vi "Check Variant Type.vi"(8 "error in (no error)":errorcluster, 10 "Variant":variant, 11 "Numeric Value in":refnum<class "Numeric Value.lvclass">) -> (0 "error out":errorcluster, 3 "Numeric Value out":refnum<class "Numeric Value.lvclass">)   [LabVIEW 2020, in "Composed Columns.lvlib" / "Numeric Value.lvclass"]
uses:
  Numeric Value.lvclass
  <vilib>/Utility/Data Type/NI_Data Type.lvlib
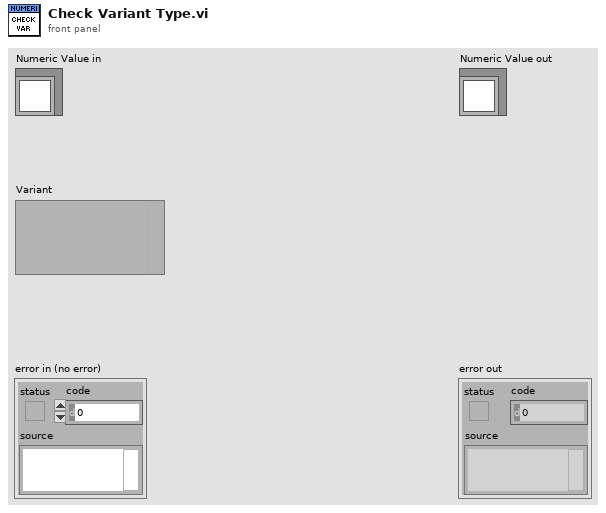
[diagram p1: front panel]
types:
  T1 = typedef "NI_Data Type.lvlib/Data Type.ctl" = enum8{"Invalid Type", "Void", "I8", "I16", "I32", "I64", "U8", "U16", "U32", "U64", "Single Float", "Double Float", "Extended Float", "Single Complex", "Double Complex", "Extended Complex", "Enum U8", "Enum U16", "Enum U32", "Enum U64", "Single Float With Unit", "Double Float With Unit", "Extended Float With Unit", "Single Complex with Unit", "Double Complex with Unit", "Extended Complex with Unit", "Boolean", "String", "Path", "Picture", "Tag", "Array", "Cluster", "Variant", "LV Variant", "Waveform", "Timestamp", "Digital Waveform", "Digital Data", "ExpressData", "Refnum", "External Data", "VI", "Poly VI", "LabVIEW Class Instance", "Fixed Point", "Set Collection", "Map Collection"}
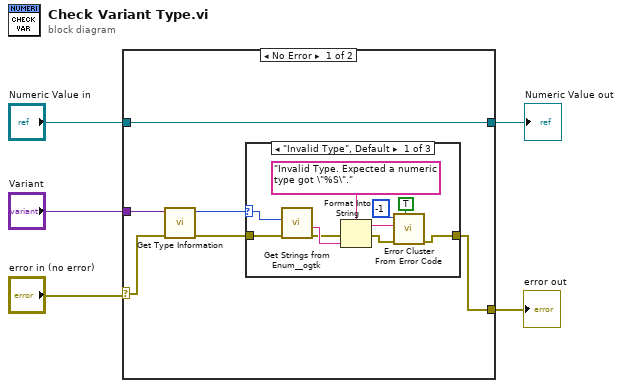
[diagram p0: block diagram]
diagram:
  n1 = case shown="No Error" "error in (no error)" {
    selector: "error in (no error)" -> [w8 w25]
    tunnel: "Variant" -> [w11 _]
    tunnel: [w6 w25] -> w3
    tunnel: "Numeric Value in" -> [w9 w24]
    tunnel: [w9 w24] -> w1
    frame No Error {
      n2 = call <vilib>:"Get Type Information.vi"("error in (no error)"=w8, "variant"=w11) -> ("error out"=w7:errorcluster, "type"=w10:T1)  [unwired: 5 in, 3 out]
      n3 = case shown="\"Invalid Type\", Default" w10 {
        selector: w10 -> [w20 _ _]
        tunnel: w7 -> [w21 w22 w23]
        tunnel: [w12 w22 w23] -> w6
        frame "Invalid Type", Default {
          n4 = call <userlib>:"Get Strings from Enum__ogtk.vi"("error in (no error)"=w21, "Enum"=w20) -> ("error out"=w17:errorcluster, "String Value"=w18:string)  [unwired: 6 in, 2 out]
          n5 = Format Into String(format string="Invalid Type. Expected a numeric type got \"%S\".", error in=w17, w18) -> (resulting string=w16:string, error out=w13:errorcluster)  [unwired: 1 in]
          n6 = call <vilib>:"Error Cluster From Error Code.vi"("show call chain? (False)"=TRUE, "error in (no error)"=w13, "error message (\"\")"=w16, "error code (0)"=-1) -> ("error out"=w12:errorcluster)  [unwired: 5 in]
        }
        frame "I8".."Extended Float" {
        }
        frame "Enum U8".."Enum U64" {
        }
      }
    }
    frame Error {
    }
  }
  "error out" <- w3
  "Numeric Value out" <- w1
